vi "Close.vi"(8 "error in (no error)":errorcluster, 11 "uService Test in":refnum<class "test_us.lvclass">) -> (0 "error out":errorcluster, 3 "uService Test out":refnum<class "test_us.lvclass">)   [LabVIEW 2026, in "test_us.lvlib" / "test_us.lvclass"]
uses:
  test_us.lvclass
  C:/LabVIEW Code/TALOS/talos/Father of all uServices/Father of all uServices/Father of all uServices.lvclass
  Father of all uServices/Father of all uServices/Children Methods/Save Waveform Chart history - single plot.vi
  C:/LabVIEW Code/TALOS/talos/Ancestor/Ancestor/Ancestor.lvclass
  C:/LabVIEW Code/TALOS/builds/Actor Framework PPL/Actor Framework.lvlibp/1abvi3w/vi.lib/ActorFramework/Actor/Actor.lvclass
  C:/LabVIEW Code/TALOS/talos/Test Stuff/test_us/test_us.lvclass
  Father of all uServices/Father of all uServices/Father of all uServices.lvclass
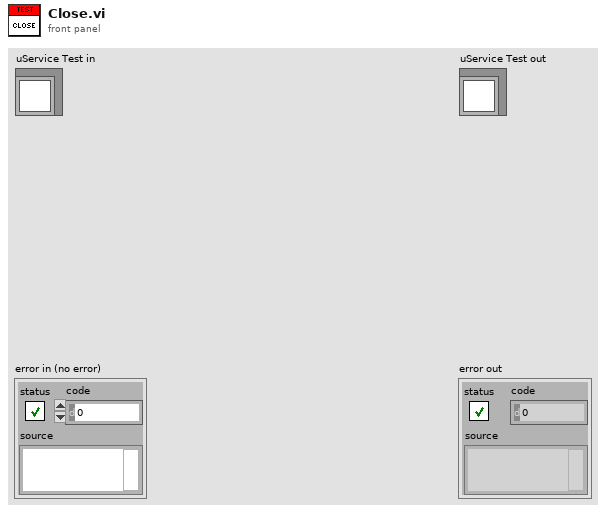
[diagram p1: front panel]
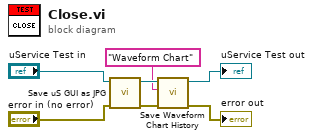
[diagram p0: block diagram]
diagram:
  n1 = call-dynamic "Save uS GUI as JPG.vi"("error in (no error)"="error in (no error)", "Father of all uServices in"="uService Test in") -> ("error out"=w3:errorcluster, "Father of all uServices out"=w5:refnum<class "test_us.lvclass">)  [unwired: 8 in]
  n2 = call-poly "Save Waveform Chart History.vi"("error in (no error)"=w3, "Plot GUI label"="Waveform Chart", "Father of all uServices in"=w5) -> ("error out"=→"error out":errorcluster, "Father of all uServices out"=→"uService Test out":refnum<class "test_us.lvclass">)  [unwired: 7 in]
